vi "Read ToD.vi"(8 "error in (no error)":errorcluster, 11 "Daily in":refnum<class "Daily.lvclass">) -> (0 "error out":errorcluster, 2 "ToD":timestamp, 3 "Daily out":refnum<class "Daily.lvclass">)   [LabVIEW 2020, in "Daily.lvclass"]
uses:
  Daily.lvclass
  Daily.lvclass/Daily.ctl
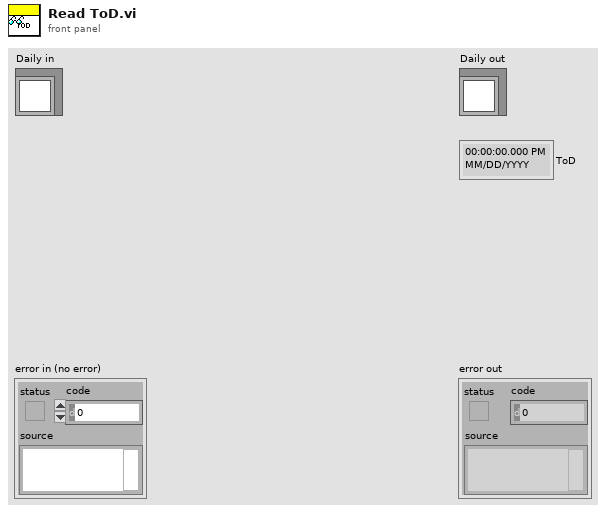
[diagram p1: front panel]
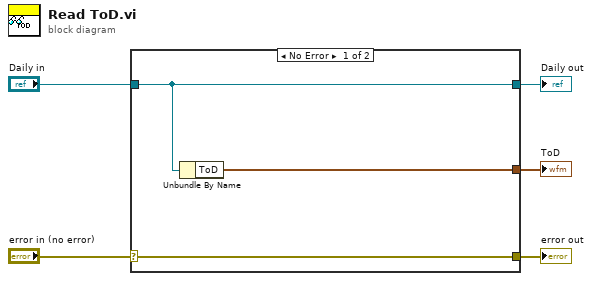
[diagram p0: block diagram]
diagram:
  n1 = case shown="No Error" "error in (no error)" {
    selector: "error in (no error)" -> [w8 w9]
    tunnel: [w8 w9] -> w4
    tunnel: [w7 w10] -> w2
    tunnel: "Daily in" -> [w7 w10]
    tunnel: [w6 _] -> w1
    frame No Error {
      n2 = Unbundle By Name(w7) -> ("ToD"=w6:timestamp)
    }
    frame Error {
    }
  }
  "error out" <- w4
  "Daily out" <- w2
  "ToD" <- w1
